vi "Query - DBL - 1D.vi"(8 "error in":errorcluster, 10 "Query":string, 11 "Module ID":i32=-1) -> (0 "error out":errorcluster, 1 "Meta Data":variant, 2 "Return Data":dbl[](array[numeric]), 4 "Field Names":string[](array[string]))   [LabVIEW 2014, in "DB_CONNECTOR.lvlib"]
uses:
  DB_CONNECTOR.lvlib
  hse-misc/Conversion/ConvertStringToFloat_Array-2D.vi
  hse-misc/hse-misc.lvlib
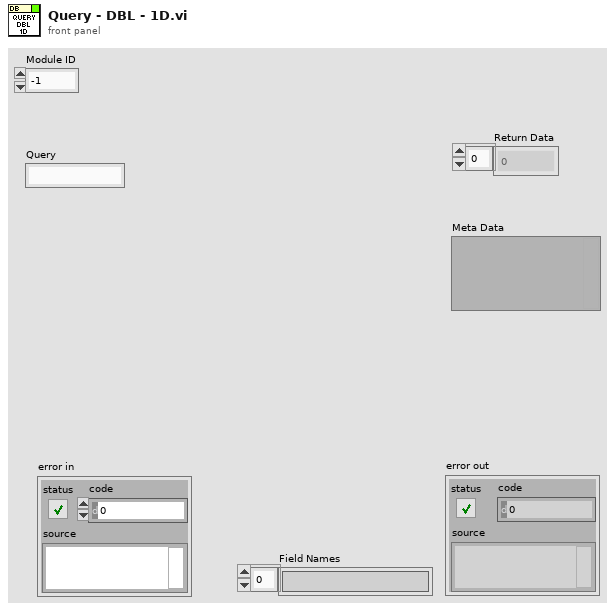
[diagram p1: front panel]
types:
  T1 = typedef "DB_CONNECTOR.lvlib/Query (Reply Payload)--cluster.ctl" = cluster{"Return Data":string[][], "Meta Data":variant, "Field Names":string[], "Query_error":errorcluster}
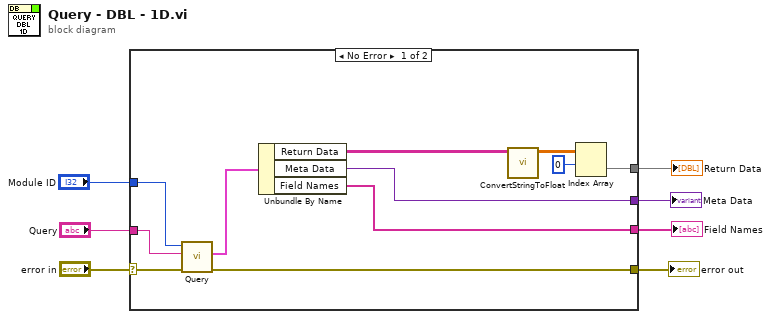
[diagram p0: block diagram]
diagram:
  n1 = case shown="No Error" "error in" {
    selector: "error in" -> [w18 w19]
    tunnel: [w13 w19] -> w6
    tunnel: "Query" -> [w16 _]
    tunnel: "Module ID" -> [w15 _]
    tunnel: [w12 _] -> w2
    tunnel: [w9 _] -> w3
    tunnel: [w8 _] -> w1
    frame No Error {
      n2 = call "Query.vi"("error in (no error)"=w18, "Query"=w16, "Module ID"=w15) -> ("error out"=w13:errorcluster, "Reply Payload"=w17:T1)  [unwired: 7 in]
      n3 = Unbundle By Name(w17) -> ("Return Data"=w14:string[][], "Meta Data"=w12:variant, "Field Names"=w8:string[])
      n4 = call-poly "ConvertStringToFloat.vi"("params"=w14) -> ("Array"=w11:dbl[][])  [unwired: 10 in]
      n5 = Index Array(array=w11, index (row)=0) -> (element=w9:dbl[])  [unwired: 1 in]
    }
    frame Error {
    }
  }
  "error out" <- w6
  "Return Data" <- w3
  "Meta Data" <- w2
  "Field Names" <- w1
